vi "Separate Chars to String.vi"(11 "Array":string[](array[string])) -> (3 "String":string)   [LabVIEW 2021]
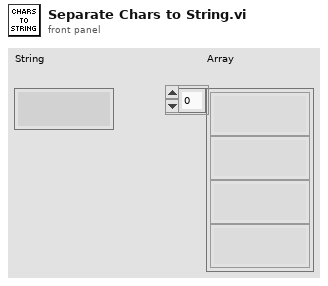
[diagram p1: front panel]
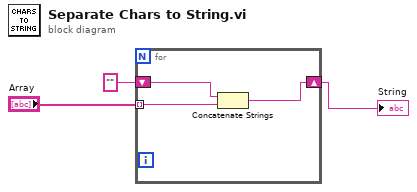
[diagram p0: block diagram]
diagram:
  n1 = for {
    tunnel: "Array" -> [w5] mode=indexing
    shift-right: [w4] -> w1
    shift-left: "" -> [w6]
    n2 = Concatenate Strings(w6, w5) -> (w4:string)
  }
  "String" <- w1
